vi "SAM.vi"(0 "System no.":i32=1 min=1 max=4 step=1, 2 "Axis":string[](array[string]), 3 "Drive States":T1[](array[typedef]), 5 "error in":errorcluster) -> (19 "error out":errorcluster)   [LabVIEW 2020]
doc: "SAM (Set Axis Mode) \n\nDescription\nSets the mode of operation for the axis.\nThe mode of operation can only be set when the axis is in the Operation enabled state. For \nfurther details, see \"Drive State Machine\" (p. 101). \n\nFormat\nSAM <AxisID> <OperationMode>\n\nArguments\n<AxisID>\nAn axis of the controller\nThe available axes can be queried with USG? SYS.\nPossible values: Alias of the axis (p. 94) \n<OperationMode>\nMode of operation of the axis \nThe permitted modes of operation can be queried with USG? PROP (p. 79). \nThe mode of operation is specified as a decimal or hexadecimal value.\nPossible values: See list of modes of operation (p. 102) \n\nResponse\nnone\n\nExample\nAxis 1 is to be operated in position control. For this purpose, the motor is first activated for the \naxis. Before the mode of operation can be set to Closed-Loop Position, the axis must also be \nreferenced. The mode of operation is specified here as a hexadecimal number (0x2).\n>>sam?\n<<AXIS_1=0x0\n<<AXIS_2=0x0\n>>eax?\n<<AXIS_1=0\n<<AXIS_2=0\n>>eax axis_1 1\n>>eax?\n<<AXIS_1=1\n<<AXIS_2=0\n>>sam?\n<<AXIS_1=0x0\n<<AXIS_2=0x0\n>>frf?\n<<AXIS_1=0\n<<AXIS_2=0\n>>err?\n<<0 - (error 0 - \"No error\")\n>>sam axis_1 0x2\n>>err?\n<<49170 - (error 49170 - \"Axis not referenced \")\n>>frf axis_1\n>>frf?\n<<AXIS_1=1\n<<AXIS_2=0\n>>sam axis_1 0x2\n>>err?\n<<0 - (error 0 - \"No error\")\n>>sam?\n<<AXIS_1=0x2\n<<AXIS_2=0x0\n\nNotes\nThe current mode of operation can be queried with the SAM? command (p. 54) and is also \ncontained in the status register of the axis (p. 97), which can be queried with the STV? \ncommand (p. 66). \n\nUser command level\nUSR"
uses:
  ModeOfOperation.ctl
panel:
  # "SAM (Set Axis Mode) \n\nSets the mode of operation for the axis.\nThe mode of operation can only be set when the axis is in the Operation enabled state. For further details, see \"Drive State Machine\"."
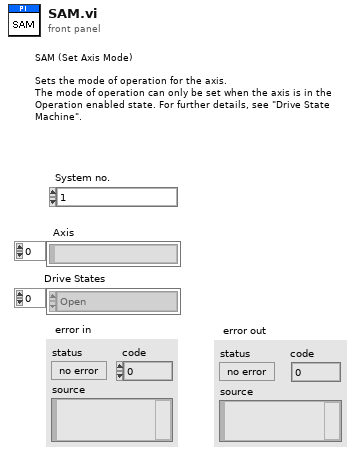
[diagram p1: front panel]
types:
  T1 = typedef "ModeOfOperation.ctl" = enum16{"Open", "Open-Loop Position", "Closed-Loop Position", "Open-Loop Velocity", "Closed-Loop Velocity", "Open-Loop Force", "Closed-Loop Force", "Step Operation"}
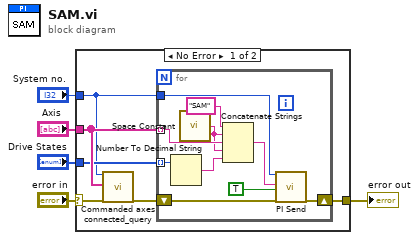
[diagram p0: block diagram]
diagram:
  n1 = case shown="No Error" "error in" {
    selector: "error in" -> [w10 w22]
    tunnel: "Drive States" -> [w7 _]
    tunnel: [w11 w22] -> w4
    tunnel: "Axis" -> [w8 _]
    tunnel: "System no." -> [w6 _]
    frame No Error {
      n2 = call "Commanded axes connected_query.vi"("System no."=w6, "Commanded axes"=w8, "error in"=w10) -> ("error out"=w9:errorcluster)  [unwired: 16 out]
      n3 = for {
        shift-right: [w21] -> w11
        shift-left: w9 -> [w20]
        tunnel: w8 -> [w15] mode=indexing
        tunnel: w7 -> [w16] mode=indexing
        tunnel: w6 -> [w12]
        n4 = Number To Decimal String(number=w16) -> (decimal integer string=w13:string)  [unwired: 1 in]
        n5 = call "Space Constant.vi"() -> ("String"=w14:string)
        n6 = Concatenate Strings("SAM", w14, w15, w14, w13) -> (w17:string)
        n7 = call "PI Send.vi"("System no."=w12, "String to send"=w17, "Attach termination char.?"=TRUE ("Attach Linefeed?"), "error in"=w20) -> ("error out"=w21:errorcluster)  [unwired: 2 in, 13 out]
      }
    }
    frame Error {
    }
  }
  "error out" <- w4
